vi "Rotation3d_UnaryMinus.vi"(11 "in Rotation3d":T1={"Q_quaternion"={"R"=1.0, "V"=[0.0, 0.0, 0.0]}}) -> (3 "out Rotation3d":T1={"Q_quaternion"={"R"=1.0, "V"=[0.0, 0.0, 0.0]}})   [LabVIEW 2019, in "Trajectory_Library.lvlib"]
doc: "Takes the inverse of the current rotation.\n\nParameters:\n - IN ROTATION3D - This ROTATION3D data structure\n\nResults:\n - OUT ROTATION3D - The negated ROTATION3D data structure."
uses:
  Trajectory_Library.lvlib
  TypeDef/QUATERNION.ctl
  TypeDef/ROTATION3D.ctl
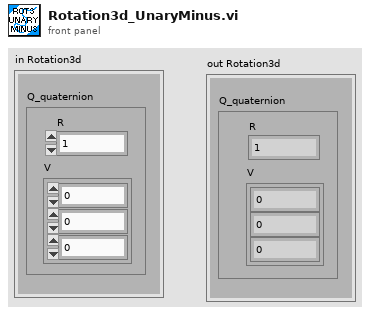
[diagram p1: front panel]
types:
  T1 = typedef "Trajectory_Library.lvlib/ROTATION3D.ctl" = cluster{"Q_quaternion":T2}
  T2 = typedef "Trajectory_Library.lvlib/QUATERNION.ctl" = cluster{"R":dbl, "V":dbl[]}
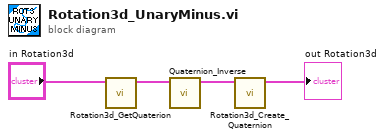
[diagram p0: block diagram]
diagram:
  n1 = call "Rotation3d_GetQuaterion.vi"("in Rotation3d"="in Rotation3d") -> ("out Quaterion"=w1:T2)  [unwired: 10 in]
  n2 = call "Quaternion_Inverse.vi"("Quaternion"=w1) -> ("Inverse"=w3:T2)  [unwired: 10 in]
  n3 = call "Rotation3d_Create_Quaternion.vi"("Quaternion"=w3) -> ("Rotation3d"=→"out Rotation3d":T1)  [unwired: 10 in]
